vi "Add Value to Database.vi"(8 "error in (no error)":errorcluster, 9 "Entry Value":string, 10 "Entry Name":string, 11 "Dictionary In":refnum<class "String Database.lvclass">=refnum) -> (0 "error out":errorcluster, 2 "replaced":bool, 3 "Dictionary Out":refnum<class "String Database.lvclass">)   [LabVIEW 2018, in "String Database.lvlib" / "String Database.lvclass"]
uses:
  String Database.lvclass
  String Database.lvclass/String Database.ctl
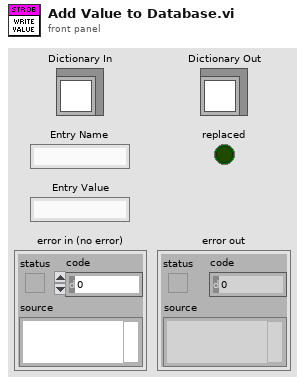
[diagram p1: front panel]
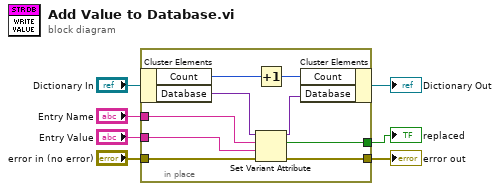
[diagram p0: block diagram]
diagram:
  n1 = in-place {
    in-place-border: "error in (no error)" -> [w16]
    in-place-border: "Entry Name" -> [w15]
    in-place-border: "Entry Value" -> [w14]
    in-place-border: [w13] -> w4
    in-place-border: [w12] -> w1
    n2 = in-place-cluster #1("Dictionary In") -> ("Count"=w8:i32, "Database"=w11:variant)
    n3 = Increment(x=w8) -> (x+1=w9:i32)
    n4 = Set Variant Attribute(Variant=w11, name=w15, value=w14, error in=w16) -> (Variant out=w10:variant, replaced=w13:bool, error out=w12:errorcluster)
    n5 = in-place-cluster #1("Count"=w9, "Database"=w10) -> (→"Dictionary Out":refnum<class "String Database.lvclass">)
  }
  "error out" <- w1
  "replaced" <- w4
